vi "Initialize Sweep Channels.vi"(8 "error in (no error)":errorcluster, 11 "Instrument.DAQ":refnum<class "Instrument.DAQ.lvclass">) -> (0 "error out":errorcluster, 3 "Instrument.DAQ out":refnum<class "Instrument.DAQ.lvclass">)   [LabVIEW 2019, in "Instrument.DAQ.lvclass"]
uses:
  Instrument.DAQ.lvclass
  Instrument.DAQ.lvclass/Instrument.DAQ.ctl
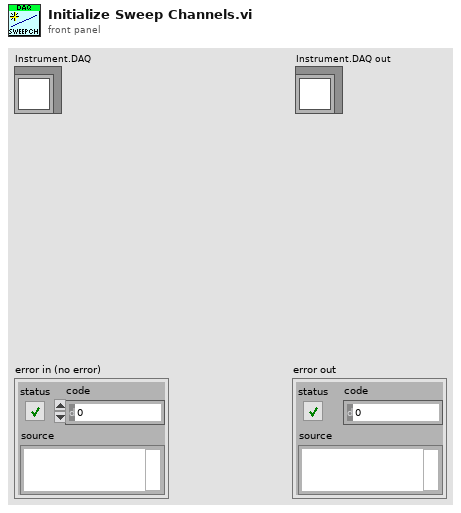
[diagram p1: front panel]
types:
  T1 = typedef "Instrument.DAQ.lvclass/Sweep.Channel--Cluster--Array.ctl" = T2[]
  T2 = typedef "Instrument.DAQ.lvclass/Sweep.Channel--Cluster.ctl" = cluster{"Enable?":bool, "Channel":u16, "Start":dbl, "End":dbl, "Pattern":T3, "Table":dbl[]}
  T3 = typedef "Instrument.DAQ.lvclass/Sweep.Pattern--Enum.ctl" = enum16{"Ramp /", "Ramp /\\", "Smooth Ramp _/", "Smooth Ramp _/\\_", "Table"}
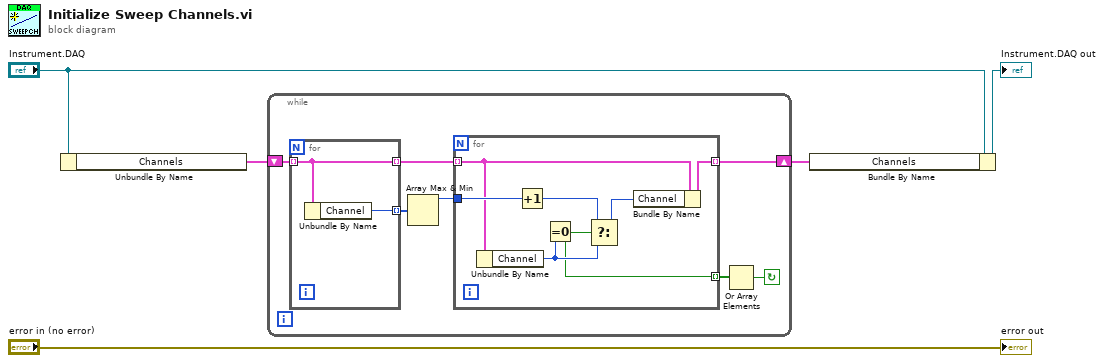
[diagram p0: block diagram]
diagram:
  n1 = Unbundle By Name("Instrument.DAQ") -> ("Channels"=w2:T1)
  n2 = while {
    shift-right: [w9] -> w1
    shift-left: w2 -> [w11]
    stop <- w6 continue-if-true
    n3 = for {
      tunnel: w11 -> [w13] mode=indexing
      tunnel: [w14] -> w12 mode=indexing
      tunnel: [w13] -> w8 mode=indexing
      n4 = Unbundle By Name(w13) -> ("Channel"=w14:u16)
    }
    n5 = Array Max & Min(array=w12) -> (max value=w10:u16)  [unwired: 3 out]
    n6 = for {
      tunnel: w8 -> [w20] mode=indexing
      tunnel: w10 -> [w21]
      tunnel: [w17] -> w9 mode=indexing
      tunnel: [w15] -> w7 mode=indexing
      n7 = Unbundle By Name(w20) -> ("Channel"=w16:u16)
      n8 = Increment(x=w21) -> (x+1=w18:u16)
      n9 = Equal To 0?(x=w16) -> (x = 0?=w15:bool)
      n10 = Select(t=w18, s=w15, f=w16) -> (s? t:f=w19:u16)
      n11 = Bundle By Name(cluster=w20, "Channel"=w19) -> (w17:T2)
    }
    n12 = Or Array Elements(Boolean array=w7) -> (logical OR=w6:bool)
  }
  n13 = Bundle By Name(cluster="Instrument.DAQ", "Channels"=w1) -> (→"Instrument.DAQ out":refnum<class "Instrument.DAQ.lvclass">)
  "error out" <- "error in (no error)"
